vi "Read explanation.vi"(11 "TestManagerMsg.Verbose in":refnum<class "TestManagerMsg.Verbose.lvclass">) -> (2 "explanation":string, 3 "TestManagerMsg.Verbose out":refnum<class "TestManagerMsg.Verbose.lvclass">)   [LabVIEW 2013, in "Caraya.lvlib" / "TestManagerMsg.Verbose.lvclass"]
uses:
  TestManagerMsg.Verbose.lvclass
  TestManagerMsg.Verbose.lvclass/TestManagerMsg.Verbose.ctl
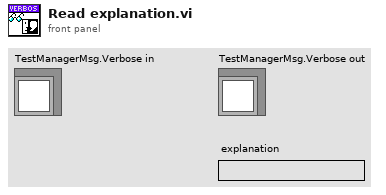
[diagram p1: front panel]
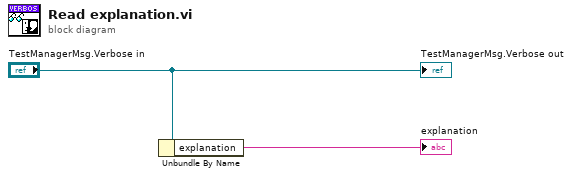
[diagram p0: block diagram]
diagram:
  n1 = Unbundle By Name("TestManagerMsg.Verbose in") -> ("explanation"=→"explanation":string)
  "TestManagerMsg.Verbose out" <- "TestManagerMsg.Verbose in"
